vi "Update AIV Values.vi"(0 "Heat Flow Results in":refnum<class "Heat Flow Results.lvclass">, 1 "R load U":dbl, 2 "I Load":dbl, 3 "P_teg":dbl, 5 "error in":errorcluster, 7 "R shunt U":dbl, 9 "I_heater":dbl, 11 "R htr U":dbl, 13 "P_heater":dbl) -> (14 "Heat Flow Results out":refnum<class "Heat Flow Results.lvclass">, 19 "error out":errorcluster)   [LabVIEW 2019, in "Results.lvlib" / "Heat Flow Results.lvclass"]
uses:
  Heat Flow Results.lvclass
  Heat Flow Results.lvclass/Heat Flow Results.ctl
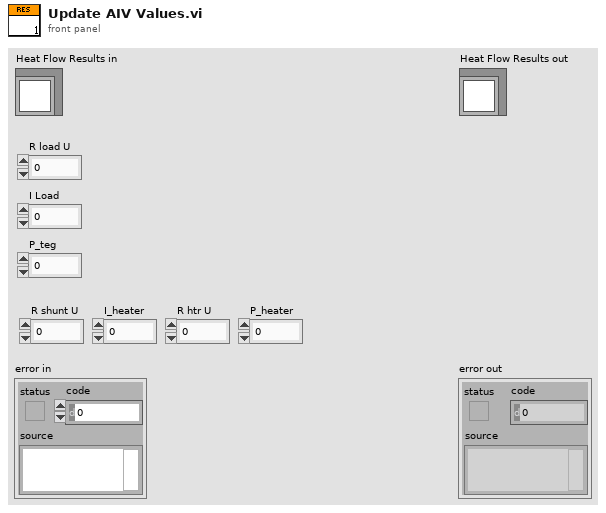
[diagram p1: front panel]
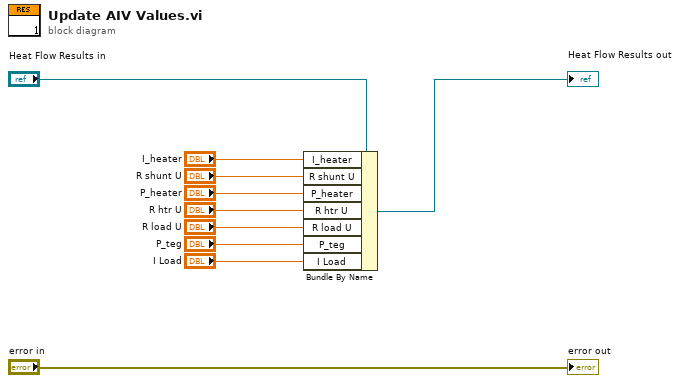
[diagram p0: block diagram]
diagram:
  n1 = Bundle By Name(cluster="Heat Flow Results in", "I_heater"="I_heater", "R shunt U"="R shunt U", "P_heater"="P_heater", "R htr U"="R htr U", "R load U"="R load U", "P_teg"="P_teg", "I Load"="I Load") -> (→"Heat Flow Results out":refnum<class "Heat Flow Results.lvclass">)
  "error out" <- "error in"
